vi "Serial Arduino Example.vi"() -> ()   [LabVIEW 2010]
uses:
  <vilib>/express/express analysis/Spectral/XNode/ExpressSpectralMeasurementsBlockNode.xnode
  <vilib>/Instr/_visa.llb/VISA Configure Serial Port (Instr).vi
  <vilib>/express/express analysis/Spectral/Block/exnSpectralBlock spectral measurements power poly.vi
  <vilib>/express/express analysis/Spectral/Block/exnSpectralBlock spectral measurements power DDT.vi
panel:
  out "Power Spectrum":dynamicdata(graph)
  out "Waveform Chart":dynamicdata(graph)
  out "Serial Values":dbl
  out "Voltage":dbl
  out "Actual Bytes read":dbl
  in  "Bytes to read":dbl
  in  "stop":bool
  in  "flow control":u16(ring) items=["None"=0, "XON/XOFF"=1, "RTS/CTS"=2, "DTR/DSR"=4]
  in  "stop bits":u16(ring)=10 items=["1.0"=10, "1.5"=15, "2.0"=20]
  in  "parity":u16(ring) items=["None", "Odd", "Even", "Mark", "Space"]
  in  "data bits":u16=8 min=5 max=8 step=1
  in  "VISA resource name":refnum<visa-resource-name>="COM1"
  in  "baud rate":u32=9600
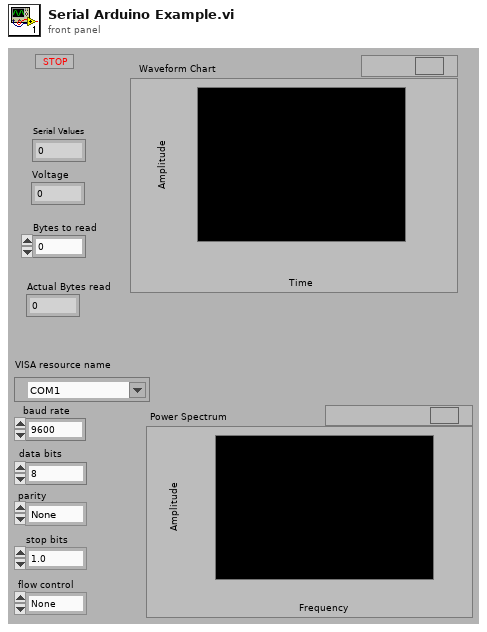
[diagram p1: front panel]
types:
  T1 = cluster{"averaging mode":u16, "weighting mode":u16, "number of averages":u32}
  T2 = cluster{"dB On (F)":bool, "unwrap phase (F)":bool, "convert to degree (F)":bool}
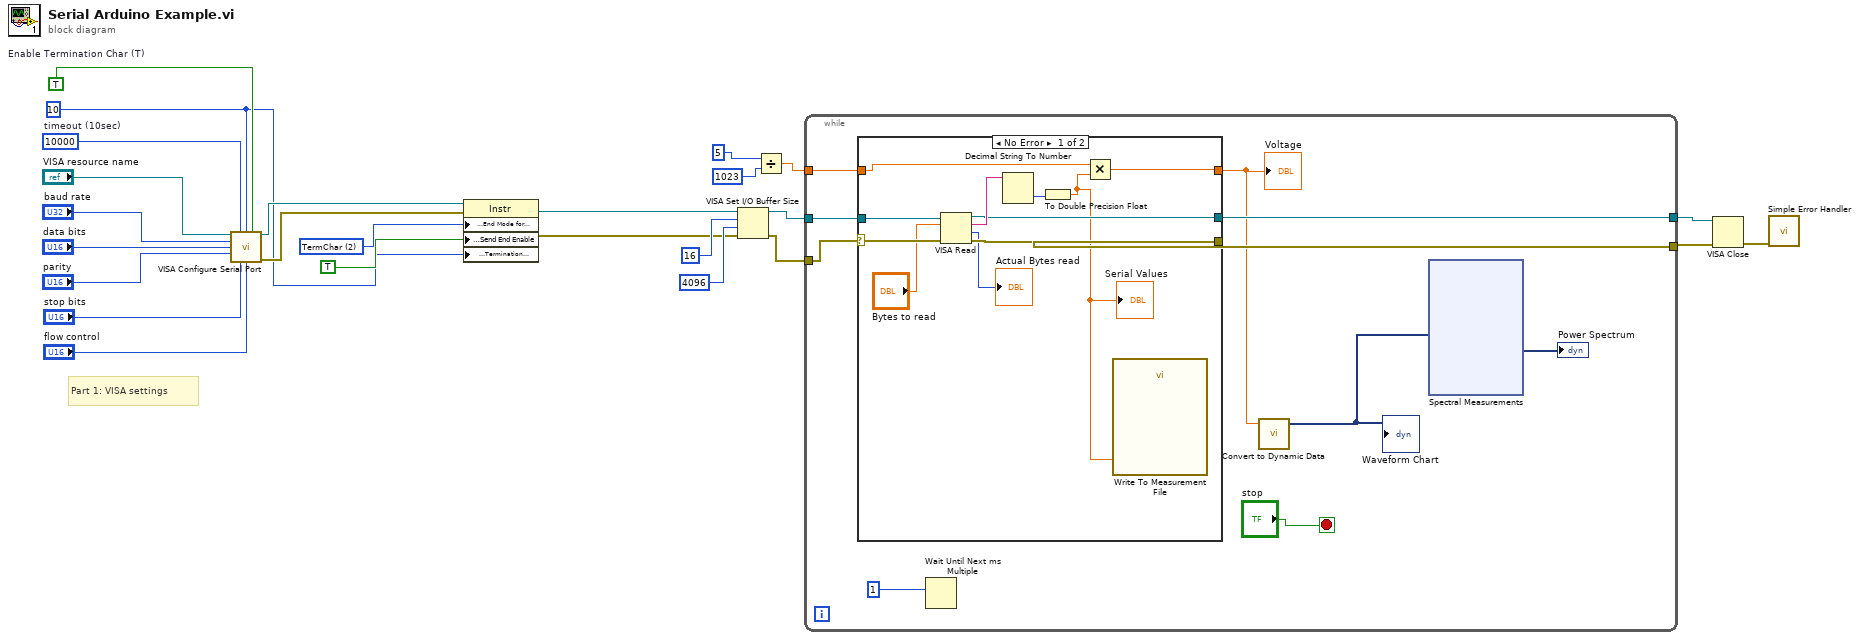
[diagram p0: block diagram]
diagram:
  w17 = u16 2 items=["None", "LastBit", "TermChar", "Break"] ("Serial Settings:Serial End Mode for Writes")
  w13 = u8 10
  w21 = TRUE  # Enable Termination Char (T)
  w22 = u32 10000  # timeout (10sec)
  # "Part 1: VISA settings"
  n1 = call-poly "VISA Configure Serial Port"("VISA resource name"="VISA resource name", "timeout (10sec)"=w22, "termination char\n(0xA = '\\n' = LF)"=w13, "Enable Termination\nChar (T)"=w21, "baud rate (9600)"="baud rate", "data bits (8)"="data bits", "parity (0:none)"="parity", "stop bits (10: 1 bit)"="stop bits", "flow control (0:none)"="flow control") -> ("VISA resource name out"=w16:refnum<visa-resource-name>, "error out"=w15:errorcluster)  [unwired: 1 in, 4 out]
  n2 = property class="Instr"(reference=w16, error in=w15, "Serial Settings:End Mode for Writes"=w17, "Message Based Settings:Send End Enable"=TRUE, "Message Based Settings:Termination Character"=w13) -> (reference out=w10:refnum<visa-resource-name>, error out=w1:errorcluster)
  n3 = VISA Set I/O Buffer Size(VISA resource name=w10, mask (16)=16, size (4096)=4096, error in (no error)=w1) -> (VISA resource name out=w9:refnum<visa-resource-name>, error out=w8:errorcluster)
  n4 = Divide(x=5, y=1023) -> (x/y=w6:dbl)
  n5 = while {
    tunnel: w9 -> [w33]
    tunnel: w8 -> [w35]
    tunnel: w6 -> [w34]
    tunnel: [w32] -> w4
    tunnel: [w30] -> w3
    stop <- "stop" stop-if-true
    n6 = case shown="No Error" w35 {
      selector: w35 -> [w55 w57]
      tunnel: w34 -> [w48 w56]
      tunnel: w33 -> [w54 w58]
      tunnel: [w52 w58] -> w32
      tunnel: [w51 w57] -> w30
      tunnel: [w46 w56] -> w28
      frame No Error {
        n7 = VISA Read(VISA resource name=w54, byte count="Bytes to read", error in (no error)=w55) -> (VISA resource name out=w52:refnum<visa-resource-name>, read buffer=w53:string, return count=→"Actual Bytes read":u32, error out=w51:errorcluster)
        n8 = Decimal String To Number(string=w53) -> (number=w47:i32)  [unwired: 1 in, 2 out]
        n9 = To Double Precision Float(number=w47) -> (double precision float=w45:dbl)
        "Serial Values" <- w45
        n10 = Multiply(x=w48, y=w45) -> (x*y=w46:dbl)
        n11 = call "Write To Measurement File"("Signals"=w45) -> ()  [unwired: 16 in, 3 out]
      }
      frame Error {
      }
    }
    "Voltage" <- w28
    n12 = Wait Until Next ms Multiple(millisecond multiple=1) -> ()  [unwired: 1 out]
    n13 = call "Convert to Dynamic Data"("Double"=w28) -> ("Dynamic Data Type"=w27:dynamicdata)  [unwired: 3 in]
    "Waveform Chart" <- w27
    n14 = xnode "Spectral Measurements"("Signals"=w27) -> ("Power Spectrum"=→"Power Spectrum":dynamicdata)  [unwired: 1 in, 1 out]
  }
  n15 = VISA Close(VISA resource name=w4, error in (no error)=w3) -> (error out=w2:errorcluster)
  n16 = call <vilib>:"Simple Error Handler.vi"("error in (no error)"=w2) -> ()  [unwired: 1 in, 8 out]
